vi "Preset subsystems.vi"(10 "appended array":bool[](array[boolean]), 11 "Enum":T1(ring)=enum."Low Hatch") -> ()   [LabVIEW 2019]
uses:
  5daef287-ccd4-4bc1-8e60-40fa11514e16.vi
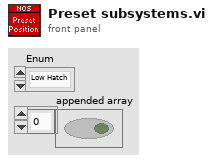
[diagram p1: front panel]
types:
  T1 = enum16{"Pick Up Ball", "Pick Up Hatch", "Shoot Ball", "Shoot Hatch", "Low Ball", "Middle Ball", "High Ball", "High Hatch", "Middle Hatch", "Low Hatch", "Cargo Ball", "Ball Loading Station", "Ball Ground", "Reserve"}
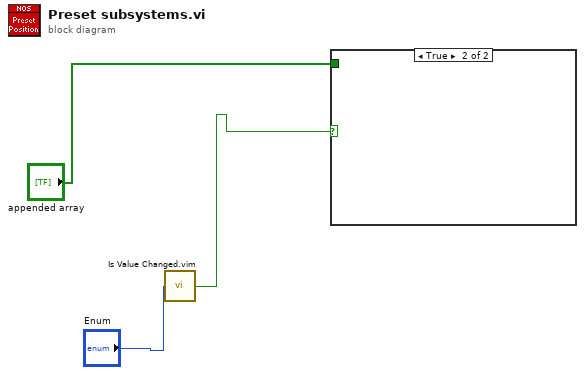
[diagram p0: block diagram]
diagram:
  n1 = call "Is Value Changed.vim"("value"="Enum") -> ("changed or first call?"=w2:bool)
  n2 = case shown="True" w2 {
    tunnel: "appended array" -> [_ _]
    frame False {
    }
    frame True {
    }
  }
